vi "replace_instances.vi"(6 "id (unnamed)":string, 8 "error in (no error)":errorcluster, 9 "instances":set{refnum<data-value>}(c389), 10 "Base Class (LabVIEW Object)":refnum<class>, 11 "Mapped Lookup in":refnum<class "Mapped Lookup.lvclass">) -> (0 "error out":errorcluster, 3 "Mapped Lookup out":refnum<class "Mapped Lookup.lvclass">)   [LabVIEW 2019, in "Lookup API.lvlib" / "Mapped Lookup.lvclass"]
uses:
  Mapped Lookup.lvclass
  Mapped Lookup.lvclass/Mapped Lookup.ctl
  <vilib>/Utility/miscctls.llb/LVMapReplaceAction.ctl
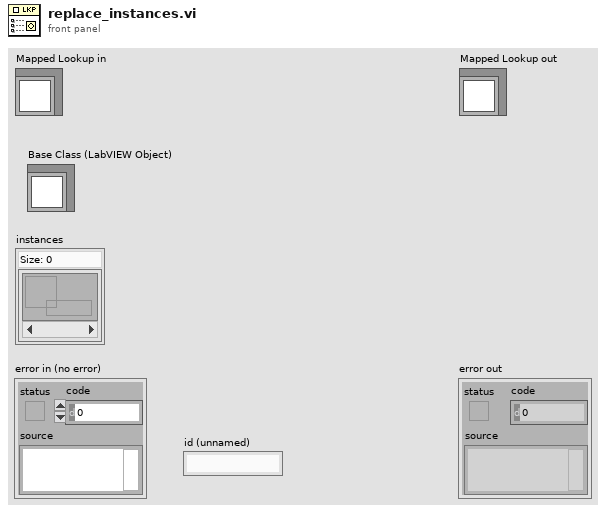
[diagram p1: front panel]
types:
  T1 = typedef "LVMapReplaceAction.ctl" = enum32{"Modify Entry only if found", "Add or Modify Entry", "Delete Entry"}
  T2 = map{string, cluster{"instances":refnum<data-value>, "events":refnum<data-value>}}
  T3 = cluster{"instances":refnum<data-value>, "events":refnum<data-value>}
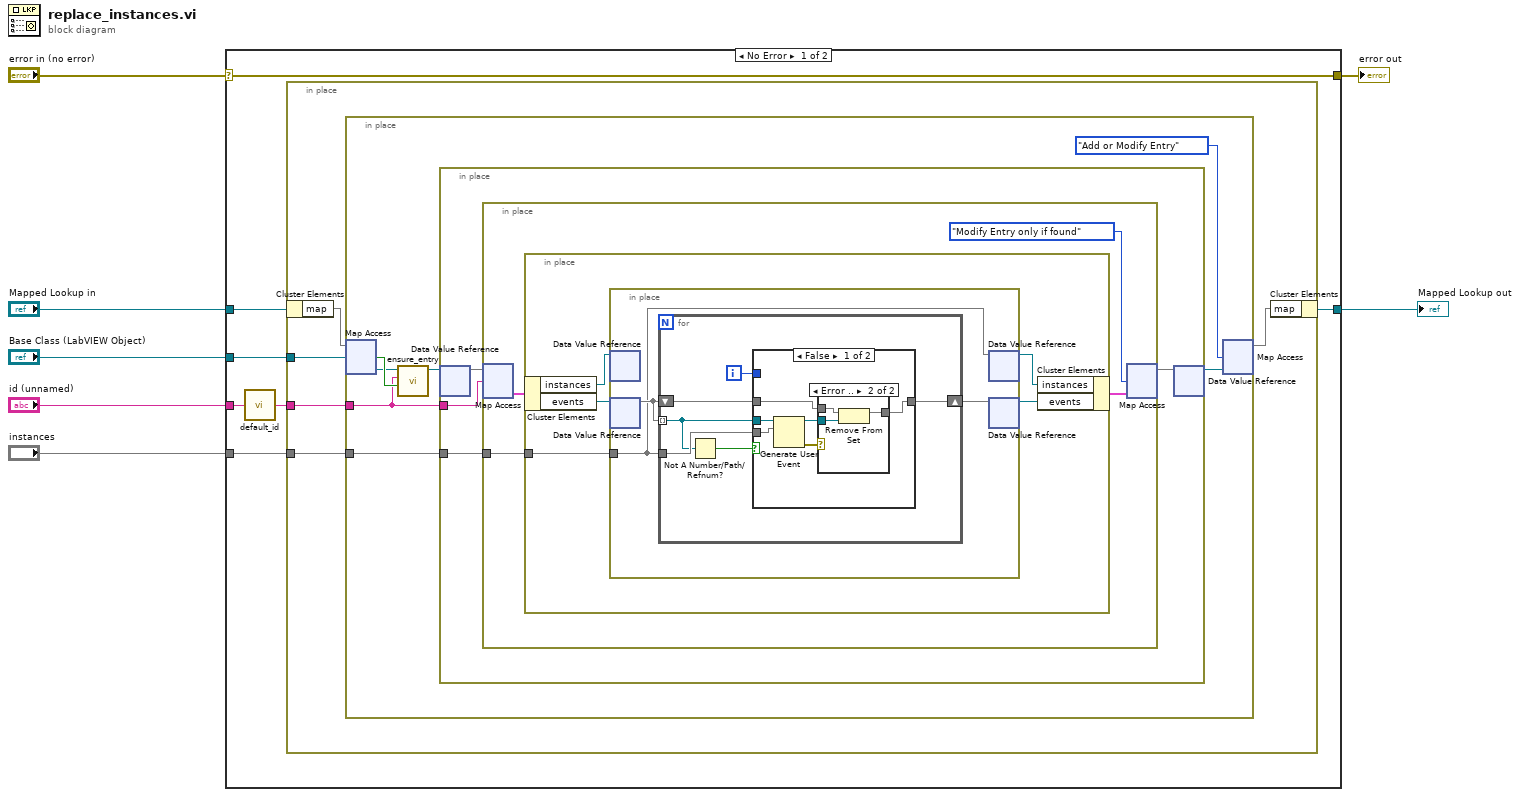
[diagram p0: block diagram]
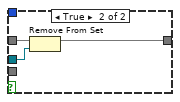
[diagram p3: hidden frame]
diagram:
  n1 = case shown="No Error" "error in (no error)" {
    selector: "error in (no error)" -> [w14 w63]
    tunnel: [w14 w63] -> w5
    tunnel: [w8 w62] -> w4
    tunnel: "Mapped Lookup in" -> [w13 w62]
    tunnel: "Base Class (LabVIEW Object)" -> [w12 _]
    tunnel: "id (unnamed)" -> [w11 _]
    tunnel: "instances" -> [w9 _]
    frame No Error {
      n2 = call "default_id.vi"("id (unnamed)"=w11) -> ("String"=w10:string)
      n3 = in-place {
        in-place-border: w12 -> [w15]
        in-place-border: w10 -> [w19]
        in-place-border: w9 -> [w18]
        n4 = in-place-cluster #1(w13) -> ("map"=w17:map{refnum<class>, refnum<data-value>})
        n5 = in-place {
          in-place-border: w19 -> [w21]
          in-place-border: w18 -> [w24]
          n6 = in-place-map #2(w17, w15) -> (w23:refnum<data-value>, w25:bool)  [unwired: 1 in]
          n7 = call "ensure_entry.vi"("not found?"=w25, "id"=w21, "named entries in"=w23) -> ("named entries out"=w22:refnum<data-value>)  [unwired: 8 in]
          n8 = in-place {
            in-place-border: w24 -> [w30]
            in-place-border: w21 -> [w28]
            n9 = in-place-dvr #3(w22) -> (w29:T2)  [unwired: 1 out]
            n10 = in-place {
              in-place-border: w30 -> [w34]
              n11 = in-place-map #4(w29, w28) -> (w33:T3)  [unwired: 1 in, 1 out]
              n12 = in-place {
                in-place-border: w34 -> [w39]
                n13 = in-place-cluster #5(w33) -> ("instances"=w38:refnum<data-value>, "events"=w36:refnum<data-value>)
                n14 = in-place {
                  in-place-border: w39 -> [w40]
                  n15 = in-place-dvr #6(w38) -> ()  [unwired: 2 out]
                  n16 = in-place-dvr #7(w36) -> (w42:set{refnum<user-event>})  [unwired: 1 out]
                  n17 = for {
                    tunnel: w40 -> [w48]
                    tunnel: w42 -> [w47] mode=indexing
                    shift-right: [w43] -> w41
                    shift-left: w42 -> [w44]
                    i -> [w45]
                    n18 = Not A Number/Path/Refnum?(number/path/refnum=w47) -> (NaN/Path/Refnum?=w46:bool)
                    n19 = case shown="False" w46 {
                      tunnel: w48 -> [w54 _]
                      tunnel: w47 -> [w53 w60]
                      tunnel: w45 -> [_ _]
                      tunnel: w44 -> [w51 w61]
                      tunnel: [w50 w59] -> w43
                      frame False {
                        n20 = Generate User Event(user event=w53, event data cluster=w54) -> (user event out=w49:refnum<user-event>, error out=w52:errorcluster)  [unwired: 2 in]
                        n21 = case shown="Error .." w52 {
                          tunnel: w51 -> [w55 w58]
                          tunnel: [w55 w57] -> w50
                          tunnel: w49 -> [_ w56]
                          frame No Error {
                          }
                          frame Error {
                            n22 = Remove From Set(10:w56, 11:w58) -> (3:w57:set{refnum<user-event>})  [unwired: 1 out]
                          }
                        }
                      }
                      frame True {
                        n23 = Remove From Set(10:w60, 11:w61) -> (3:w59:set{refnum<user-event>})  [unwired: 1 out]
                      }
                    }
                  }
                  n24 = in-place-dvr #6(w40) -> (w37:refnum<data-value>)  [unwired: 1 out]
                  n25 = in-place-dvr #7(w41) -> (w35:refnum<data-value>)  [unwired: 1 out]
                }
                n26 = in-place-cluster #5("instances"=w37, "events"=w35) -> (w32:T3)
              }
              n27 = in-place-map #4(w32, LVMapReplaceAction."Modify Entry only if found" ("action")) -> (w27:T2)  [unwired: 2 out]
            }
            n28 = in-place-dvr #3(w27) -> (w20:refnum<data-value>)  [unwired: 1 out]
          }
          n29 = in-place-map #2(w20, LVMapReplaceAction."Add or Modify Entry" ("action")) -> (w16:map{refnum<class>, refnum<data-value>})  [unwired: 2 out]
        }
        n30 = in-place-cluster #1("map"=w16) -> (w8:refnum<class "Mapped Lookup.lvclass">)
      }
    }
    frame Error {
    }
  }
  "error out" <- w5
  "Mapped Lookup out" <- w4
